vi "DAQ_trigger_control_PN.vi"(1 "Action":u8(ring) items=["OUT LOW", "OUT HIGH", "IN READ"]) -> (2 "Action success?":bool, 3 "IN state (after IN READ action only)":u8, 4 "Error out":errorcluster)   [LabVIEW 2022 SP3]
uses:
  <vilib>/Instr/_visa.llb/VISA Open Access Mode.ctl
  Globals/Meas_global.vi
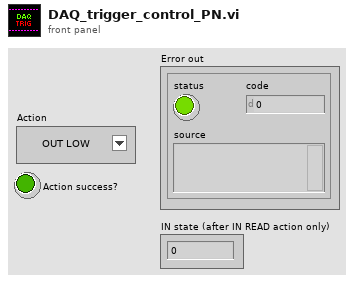
[diagram p1: front panel]
types:
  T1 = typedef "VISA Open Access Mode.ctl" = u32
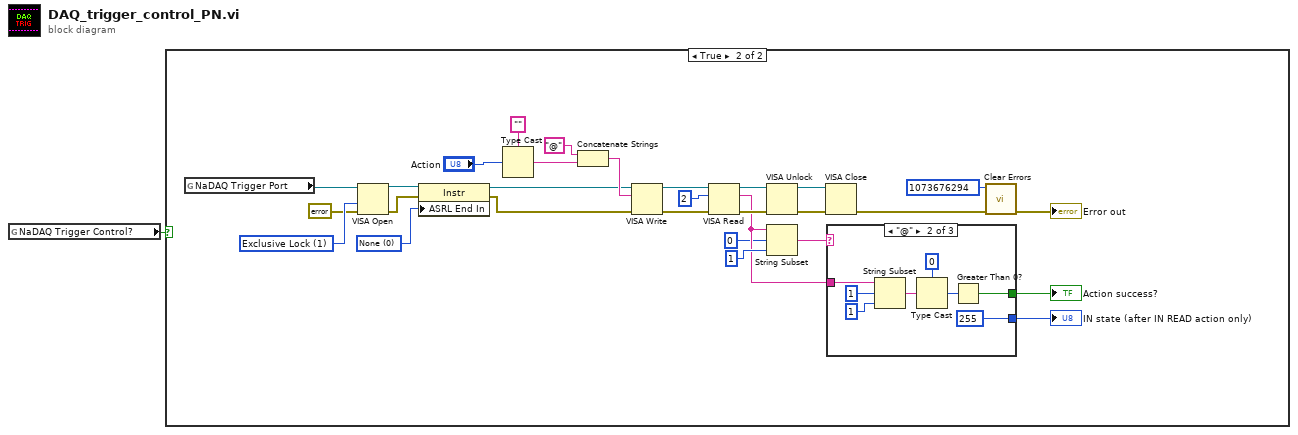
[diagram p0: block diagram]
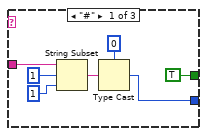
[diagram p3: hidden frame]
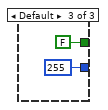
[diagram p4: hidden frame]
diagram:
  n1 = global read "Meas_global.vi" "NaDAQ Trigger Control?"() -> (w1:bool)
  n2 = case shown="True" w1 {
    frame False {
    }
    frame True {
      w28 = u16 0 items=["None", "Last Bit", "TermChar"] ("Serial Settings:End Mode for Reads")
      w30 = T1 1 items=["VISA Defaults"=0, "Exclusive Lock"=1, "Load Configured Settings"=4] ("Access Mode")
      n3 = global read "Meas_global.vi" "NaDAQ Trigger Port"() -> (w2:refnum<visa-resource-name>)
      n4 = VISA Open(access mode=w30, error in (no error)=errorcluster {"status"=FALSE, "code"=0, "source"=""}, VISA resource name=w2) -> (VISA resource name=w26:refnum<visa-resource-name>, error out=w27:errorcluster)  [unwired: 2 in]
      n5 = property class="Instr"(reference=w26, error in=w27, "ASRL End In"=w28) -> (reference out=w20:refnum<visa-resource-name>, error out=w19:errorcluster)
      n6 = Type Cast(type="", x="Action") -> (*(type *) &x=w21:string)
      n7 = Concatenate Strings("@", w21) -> (w25:string)
      n8 = VISA Write(VISA resource name=w20, write buffer=w25, error in (no error)=w19) -> (VISA resource name out=w18:refnum<visa-resource-name>, error out=w17:errorcluster)  [unwired: 1 out]
      n9 = VISA Read(VISA resource name=w18, byte count=u32 2, error in (no error)=w17) -> (VISA resource name out=w13:refnum<visa-resource-name>, read buffer=w9:string, error out=w12:errorcluster)  [unwired: 1 out]
      n10 = VISA Unlock(8:w12, 11:w13) -> (0:w14:errorcluster, 3:w15:refnum<visa-resource-name>)
      n11 = String Subset(string=w9, offset (0)=0, length (rest)=1 ("length (rest)")) -> (substring=w10:string)
      n12 = VISA Close(VISA resource name=w15, error in (no error)=w14) -> (error out=w4:errorcluster)
      n13 = case shown="\"@\"" w10 {
        tunnel: w9 -> [w37 w45 _]
        tunnel: [w32 u8 255 ("length (rest)") u8 255 ("length (rest)")] -> w7
        tunnel: [TRUE w39 FALSE] -> w6
        frame "#" {
          n14 = String Subset(string=w37, offset (0)=1, length (rest)=1 ("length (rest)")) -> (substring=w34:string)
          n15 = Type Cast(type=u8 0 ("length (rest)"), x=w34) -> (*(type *) &x=w32:u8)
        }
        frame "@" {
          n16 = String Subset(string=w45, offset (0)=1, length (rest)=1 ("length (rest)")) -> (substring=w42:string)
          n17 = Type Cast(type=u8 0 ("length (rest)"), x=w42) -> (*(type *) &x=w40:u8)
          n18 = Greater Than 0?(x=w40) -> (x > 0?=w39:bool)
        }
        frame Default {
        }
      }
      "IN state (after IN READ action only)" <- w7
      "Action success?" <- w6
      n19 = call <vilib>:"Clear Errors.vi"("error in (no error)"=w4, "specific error code to clear (0: all)"=1073676294) -> ("error out"=→"Error out":errorcluster)  [unwired: 4 in, 1 out]
    }
  }
